vi "fill_elements_strict.vi"(7 "little-endian arrays (T)":bool=TRUE, 8 "error in (no error)":errorcluster, 10 "arrayOfElements":T1[](array[typedef]), 11 "dataType in":variant) -> (0 "error out":errorcluster, 3 "dataType out":variant)   [LabVIEW 2015, in "BSON_convertors_Library.lvlib"]
doc: "Created by Artem Shevelev\nLabVIEW Portal profile: http://www.labviewportal.org/memberlist.php?mode=viewprofile&u=2340\ne-mail: artem.sh@gmail.com\nshevelev.pro"
uses:
  BSON_convertors_Library.lvlib
  typedefs/BSONelement.ctl
  typedefs/dataType.ctl
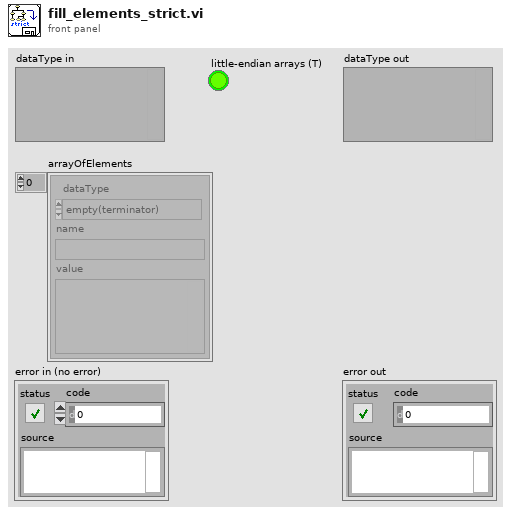
[diagram p1: front panel]
types:
  T1 = typedef "BSON_convertors_Library.lvlib/BSONelement.ctl" = cluster{"dataType":T2, "name":string, "value":variant}
  T2 = typedef "BSON_convertors_Library.lvlib/dataType.ctl" = enum8{"empty(terminator)", "double", "string", "document", "array", "binary", "Deprecated(Undefined)", "ObjectId", "boolean", "UTC datetime", "Null value", "cstring", "Deprecated(DBPointer)", "JavaScript", "Deprecated(Symbol)", "code_w_s", "int32", "uint64", "int64", "ext (decimal128)", "Min key", "Max key"}
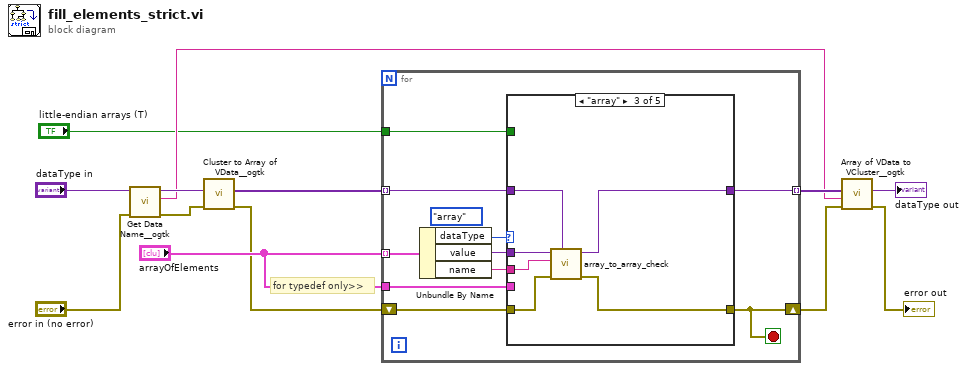
[diagram p0: block diagram]
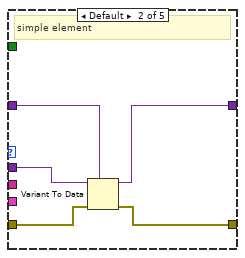
[diagram p3: hidden frame]
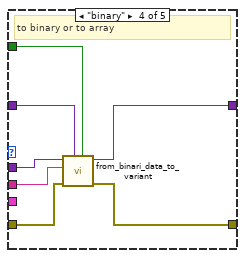
[diagram p4: hidden frame]
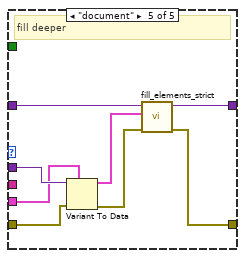
[diagram p5: hidden frame]
diagram:
  # "for typedef only>>"
  n1 = call <userlib>:"Get Data Name__ogtk.vi"("error in (no error)"="error in (no error)", "Data"="dataType in") -> ("error out"=w6:errorcluster, "Data Name"=w5:string, "Data dup"=w8:variant)  [unwired: 7 in]
  n2 = call <userlib>:"Cluster to Array of VData__ogtk.vi"("error in (no error)"=w6, "Cluster"=w8) -> ("error out"=w12:errorcluster, "Array of VData"=w11:variant[])  [unwired: 8 in]
  n3 = for {
    tunnel: "arrayOfElements" -> [w23] mode=indexing
    shift-right: [w19] -> w3
    shift-left: w12 -> [w20]
    tunnel: "arrayOfElements" -> [w18]
    tunnel: w11 -> [w17] mode=indexing
    tunnel: [w16] -> w10 mode=indexing
    tunnel: "little-endian arrays (T)" -> [w15]
    stop <- w19 stop-if-true
    (unwired) dataType."array" ("dataType")
    n4 = Unbundle By Name(w23) -> ("dataType"=w22:T2, "value"=w21:variant, "name"=w14:string)
    n5 = case shown="\"array\"" w22 {
      tunnel: w21 -> [_ w30 w31 w39 w51]
      tunnel: w20 -> [w25 w29 w36 w43 w44]
      tunnel: [w25 w26 w35 w42 w45] -> w19
      tunnel: w18 -> [_ _ _ _ w50]
      tunnel: w17 -> [w24 w28 w33 w38 w49]
      tunnel: [w24 w27 w34 w41 w46] -> w16
      tunnel: w15 -> [_ _ _ w40 _]
      tunnel: w14 -> [_ _ w32 w37 _]
      frame "empty(terminator)" {
      }
      frame Default {
        # "simple element"
        n6 = Variant To Data(error in=w29, type=w28, Variant=w30) -> (data=w27:variant, error out=w26:errorcluster)
      }
      frame "array" {
        n7 = call "array_to_array_check.vi"("dataType"=w33, "error in (no error)"=w36, "name"=w32, "value in"=w31) -> ("error out"=w35:errorcluster, "value out"=w34:variant)  [unwired: 6 in]
      }
      frame "binary" {
        # "to binary or to array"
        n8 = call "from_binari_data_to_variant.vi"("little-endian"=w40, "dataType"=w38, "error in (no error)"=w43, "name"=w37, "binaryData"=w39) -> ("error out"=w42:errorcluster, "dataOut"=w41:variant)  [unwired: 5 in]
      }
      frame "document" {
        # "fill deeper"
        n9 = Variant To Data(error in=w44, type=w50, Variant=w51) -> (data=w48:T1[], error out=w47:errorcluster)
        n10 = call "fill_elements_strict.vi"("error in (no error)"=w47, "arrayOfElements"=w48, "dataType in"=w49) -> ("error out"=w45:errorcluster, "dataType out"=w46:variant)  [unwired: 7 in]
      }
    }
  }
  n11 = call <userlib>:"Array of VData to VCluster__ogtk.vi"("error in (no error)"=w3, "Cluster Name"=w5, "Array"=w10) -> ("error out"=→"error out":errorcluster, "VCluster"=→"dataType out":variant)  [unwired: 7 in]
